vi "Read Protocol Settings from JSON.vi"(8 "error in":errorcluster, 11 "JSON file":string) -> (0 "error out":errorcluster, 3 "Configurations":T1)   [LabVIEW 2021]
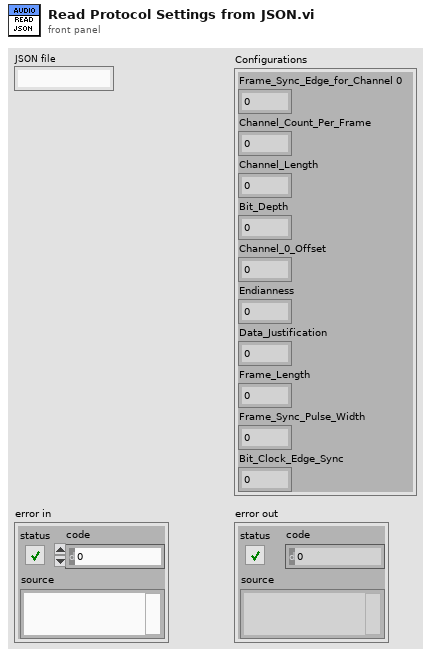
[diagram p1: front panel]
types:
  T1 = cluster{"Frame_Sync_Edge_for_Channel 0":i32, "Channel_Count_Per_Frame":i32, "Channel_Length":i32, "Bit_Depth":i32, "Channel_0_Offset":i32, "Endianness":i32, "Data_Justification":i32, "Frame_Length":i32, "Frame_Sync_Pulse_Width":i32, "Bit_Clock_Edge_Sync":i32}
  T2 = cluster{"Configurations":cluster{"Frame_Sync_Edge_for_Channel 0":i32, "Channel_Count_Per_Frame":i32, "Channel_Length":i32, "Bit_Depth":i32, "Channel_0_Offset":i32, "Endianness":i32, "Data_Justification":i32, "Frame_Length":i32, "Frame_Sync_Pulse_Width":i32, "Bit_Clock_Edge_Sync":i32}}
  T3 = enum16{"open", "replace", "create", "open or create", "replace or create", "replace or create with confirmation"}
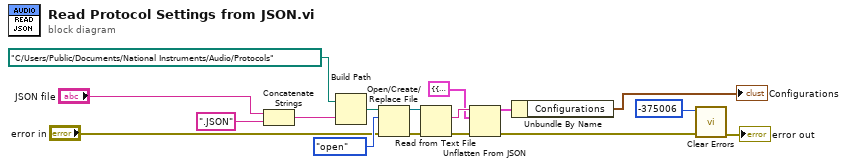
[diagram p0: block diagram]
diagram:
  n1 = Concatenate Strings("JSON file", ".JSON" ("string")) -> (w8:string)
  n2 = Build Path(base path=path "C:/Users/Public/Documents/National Instruments/Audio/Protocols", name or relative path=w8) -> (appended path=w16:path)
  n3 = Open/Create/Replace File(file path (use dialog)=w16, error in="error in", operation (0:open)=T3."open") -> (refnum out=w12:refnum<file>, error out=w14:errorcluster)  [unwired: 3 in, 1 out]
  n4 = Read from Text File(file (use dialog)=w12, error in=w14) -> (text=w11:string, error out=w13:errorcluster)  [unwired: 2 in, 2 out]
  n5 = Unflatten From JSON(JSON string=w11, type and defaults=T2 {"Configurations"={"Frame_Sync_Edge_for_Channel 0"=1, "Channel_Count_Per_Frame"=2, "Channel_Length"=32, "Bit_Depth"=24, "Channel_0_Offset"=1, "Endianness"=0, "Data_Justification"=0, "Frame_Length"=64, "Frame_Sync_Pulse_Width"=32, "Bit_Clock_Edge_Sync"=1}}, error in (no error)=w13) -> (value=w17:T2, error out=w1:errorcluster)  [unwired: 4 in]
  n6 = Unbundle By Name(w17) -> ("Configurations"=→"Configurations":T1)
  n7 = call <vilib>:"Clear Errors.vi"("error in (no error)"=w1, "specific error code to clear (0: all)"=-375006) -> ("error out"=→"error out":errorcluster)  [unwired: 4 in, 1 out]
